vi "oax_gsCascade Plot.vi"() -> ()   [LabVIEW 2017]
doc: "This is Order Analysis Toolkit demo VI."
uses:
  <vilib>/addons/Sound and Vibration/Order Analysis/Tach Process/SoundVib_TachProcess.lvlib
  <vilib>/Waveform/WDTOps.llb/WDT Waveform Duration DBL.vi
  <vilib>/addons/Sound and Vibration/Order Analysis/Resample Order Tracking/SoundVib_OrderTracking.lvlib
  <vilib>/addons/Sound and Vibration/Order Analysis/Data Presentation/SoundVib_SpectralDisplay.lvlib
  <vilib>/addons/_XControls/Waterfall Graph/SVX Waterfall Graph.xctl
panel:
  out "Cascade Plot":T1(xcontrol) caption="Waterfall Graph"
  in  "STOP":bool
  in  "Select Data":i32(listbox)=1
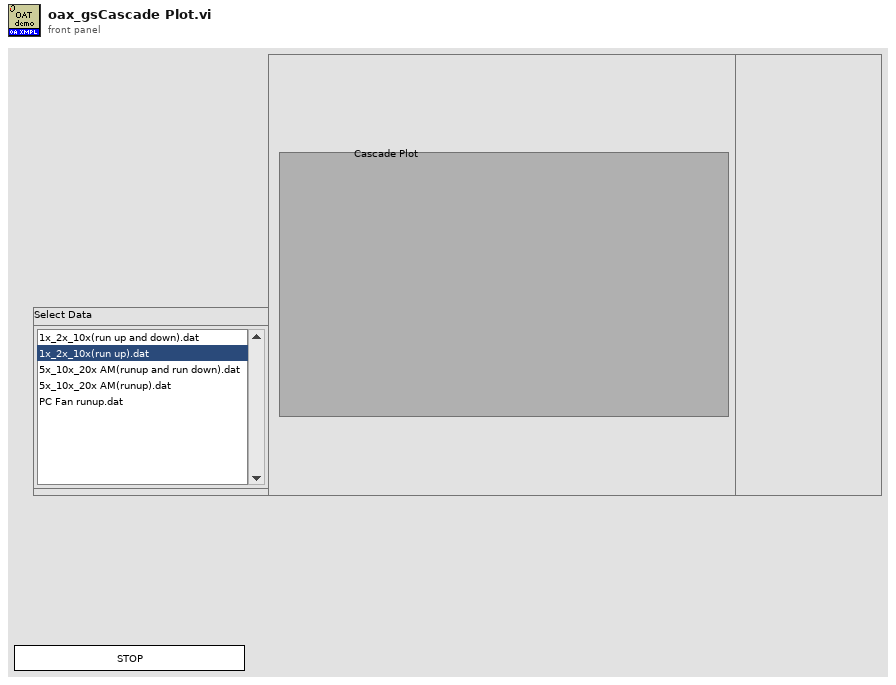
[diagram p1: front panel]
types:
  T1 = cluster{"z0":dbl, "dz":dbl, "Plots":cluster{"x0":dbl, "dx":dbl, "Y":dbl[]}[]}
  T2 = enum16{"Frequency-RPM", "RPM-Frequency", "Order-RPM", "RPM-Order"}
  T3 = typedef "SoundVib_TachProcess.lvlib/speed profile.ctl" = cluster{"time [s]":dbl[], "speed [RPM]":dbl[]}
  T4 = cluster{"z0":dbl, "dz":dbl, "waveforms":cluster{"f0":dbl, "df":dbl, "magnitude":dbl[]}[]}
  T5 = cluster{"x-axis unit label":string, "y-axis unit label":string, "z-axis unit label":string}
  T6 = cluster{"z0":dbl, "dz":dbl, "plots":cluster{"x0":dbl, "dx":dbl, "Y":dbl[]}[]}
  T7 = cluster{"pulse / rev":i32, "threshold (auto)":dbl, "slope (Rising)":u16}
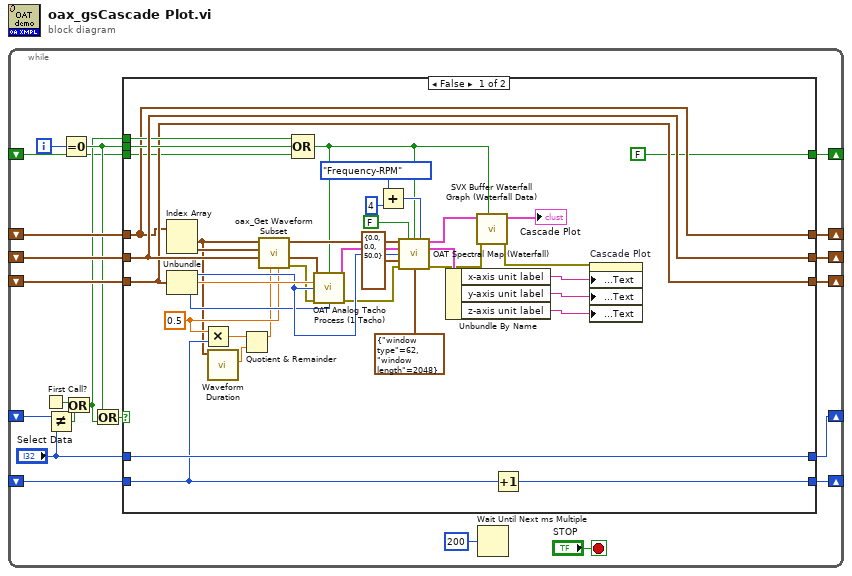
[diagram p0: block diagram]
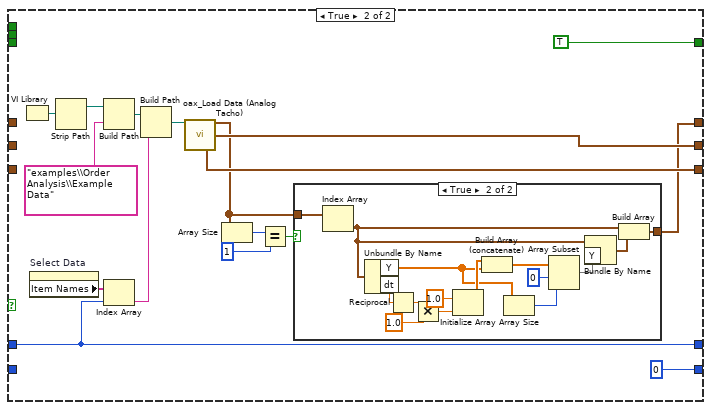
[diagram p2: hidden frame]
diagram:
  n1 = while {
    shift-right: [w17] -> _
    shift-left: _ -> [w18]
    shift-right: [w15] -> _
    shift-left: _ -> [w21]
    shift-right: [w14] -> _
    shift-left: _ -> [w19]
    shift-right: [w13] -> _
    shift-left: _ -> [w12]
    shift-right: [w3] -> _
    shift-left: _ -> [w4]
    shift-right: [w2] -> _
    shift-left: _ -> [w1]
    i -> [w11]
    stop <- "STOP" stop-if-true
    n2 = First Call?() -> (First Call?: T/F=w7:bool)
    n3 = Not Equal?(x=w18, y="Select Data") -> (x != y?=w6:bool)
    n4 = Equal To 0?(x=w11) -> (x = 0?=w10:bool)
    n5 = Or(x=w7, y=w6) -> (x .or. y?=w5:bool)
    n6 = Or(x=w10, y=w5) -> (x .or. y?=w9:bool)
    n7 = case shown="False" w9 {
      tunnel: w21 -> [w41 _]
      tunnel: w19 -> [w58 _]
      tunnel: [w59 w76] -> w17
      tunnel: "Select Data" -> [w59 w76]
      tunnel: [w41 w61] -> w15
      tunnel: [w58 w74] -> w14
      tunnel: [w52 w73] -> w13
      tunnel: w12 -> [w52 _]
      tunnel: w5 -> [w56 _]
      tunnel: w10 -> [w55 _]
      tunnel: w4 -> [w46 _]
      tunnel: [w48 0] -> w3
      tunnel: [FALSE TRUE] -> w2
      tunnel: w1 -> [w40 _]
      frame False {
        w47 = 0.5 ("y")
        n8 = Index Array(array=w41) -> (element #1=w45:waveform(dbl), element #2=w53:waveform(dbl))  [unwired: 2 in]
        n9 = Unbundle(w52) -> ("pulse / rev"=w50:i32, "threshold (auto)"=w51:dbl, "slope (Rising)"=w49:u16)
        n10 = Multiply(x=w47, y=w46) -> (x*y=w43:dbl)
        n11 = call-poly <vilib>:"Waveform Duration.vi"("waveform in"=w45) -> ("duration"=w44:dbl)  [unwired: 8 in, 2 out]
        n12 = Quotient & Remainder(x=w43, y=w44) -> (x-y*floor(x/y)=w42:dbl)  [unwired: 1 out]
        n13 = call <vilib>:"oax_Get Waveform Subset.vi"("duration"=w47, "start index"=w42, "Tach Signal"=w58, "Vibration Signal Y"=w53, "Vibration Signal X"=w45) -> ("error out"=w34:errorcluster, "Tach Signal out"=w57:waveform(dbl), "Vibration Signal X out"=w54:waveform(dbl))  [unwired: 3 in, 1 out]
        n14 = Compound Arithmetic op=OR(w56, w55, w40) -> (w24:bool)
        n15 = call <vilib>:"OAT Analog Tacho Process (1 Tacho).vi"("analog tacho signal"=w57, "reset? (F)"=w24, "threshold (auto)"=w51, "pulse/revolution (1)"=w50, "error in (no error)"=w34, "slope (Rising)"=w49) -> ("speed profile"=w60:T3, "error out"=w33:errorcluster)  [unwired: 5 in, 3 out]
        n16 = Add(x=T2."Frequency-RPM" ("plot type"), y=4) -> (x+y=w35:i32)
        n17 = call <vilib>:"OAT Spectral Map (Waterfall).vi"("scaled signal [EU]"=w54, "dB on? (F)"=FALSE ("dB on (F)"), "reset? (F)"=w24, "plot type"=w35, "speed profile"=w60, "pulse/revolution (1)"=w50, "time/speed segment [s or RPM]"=cluster{"start":dbl, "end":dbl, "step size":dbl} {"start"=0.0, "end"=0.0, "step size"=50.0} ("time/speed segment [s or rpm]"), "error in (no error)"=w33, "windows info"=cluster{"window type":u32, "window length":i32} {"window type"=62, "window length"=2048}) -> ("waterfall graph"=w26:T4, "waterfall unit labels"=w32:T5, "error out"=w23:errorcluster)  [unwired: 2 in, 2 out]
        n18 = Unbundle By Name(w32) -> ("x-axis unit label"=w31:string, "y-axis unit label"=w30:string, "z-axis unit label"=w29:string)
        n19 = call <vilib>:"SVX Buffer Waterfall Graph (Waterfall Data).vi"("reset? (F)"=w24, "error in (no error)"=w23, "waterfall graph data"=w26) -> ("error out"=w22:errorcluster, "waterfall graph data out"=→"Cascade Plot":T6)  [unwired: 7 in]
        n20 = Increment(x=w46) -> (x+1=w48:i32)
        n21 = property on="Cascade Plot"(error in=w22, "XScale.NameLbl.Text"=w31, "YScale.NameLbl.Text"=w30, "ZScale.NameLbl.Text"=w29) -> ()  [unwired: 1 in, 2 out]
      }
      frame True {
        n22 = VI Library() -> (path=w69:path)
        n23 = property on="Select Data" class="LstBox (strict)"() -> ("Item Names"=w77:string[])  [unwired: 2 in, 2 out]
        n24 = Strip Path(path=w69) -> (stripped path=w68:path)  [unwired: 1 out]
        n25 = Build Path(base path=w68, name or relative path="examples\\Order Analysis\\Example Data") -> (appended path=w72:path)
        n26 = Index Array(array=w77, index=w76) -> (element=w71:string)
        n27 = Build Path(base path=w72, name or relative path=w71) -> (appended path=w70:path)
        n28 = call <vilib>:"oax_Load Data (Analog Tacho).vi"("Data Path In"=w70) -> ("vibration data"=w62:waveform(dbl)[], "analog tacho signal"=w74:waveform(dbl), "tacho info"=w73:T7)  [unwired: 8 in, 4 out]
        n29 = Array Size(array=w62) -> (size(s)=w65:i32)
        n30 = Equal?(x=w65, y=1) -> (x = y?=w63:bool)
        n31 = case shown="True" w63 {
          tunnel: w62 -> [w78 w93]
          tunnel: [w78 w92] -> w61
          frame False {
          }
          frame True {
            n32 = Index Array(array=w93) -> (element=w91:waveform(dbl))  [unwired: 1 in]
            n33 = Unbundle By Name(w91) -> ("Y"=w80:dbl[], "dt"=w89:dbl)
            n34 = Reciprocal(x=w89) -> (1/x=w88:dbl)
            n35 = Multiply(x=w88, y=1.0) -> (x*y=w86:dbl)
            n36 = Initialize Array(1.0 ("element"), w86) -> (w82:dbl[])
            n37 = Build Array (concatenate)(w82, w80) -> (w84:dbl[])
            n38 = Array Size(array=w80) -> (size(s)=w81:i32)
            n39 = Array Subset(array=w84, index=0, length=w81) -> (w79:dbl[])
            n40 = Bundle By Name(cluster=w91, "Y"=w79) -> (w90:waveform(dbl))
            n41 = Build Array(w91, w90) -> (w92:waveform(dbl)[])
          }
        }
      }
    }
    n42 = Wait Until Next ms Multiple(millisecond multiple=u32 200) -> ()  [unwired: 1 out]
  }
